vi "mod_control changed.vi"   [LabVIEW 2020, in "niAMT.lvlib"]
uses:
  <vilib>/addons/Modulation/niAMT.lvlib
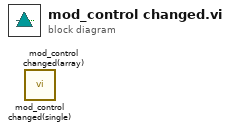
[diagram p0: block diagram]
diagram:
  n1 = call <vilib>:"mod_control changed(single).vi"() -> ()  [unwired: 9 in, 1 out]
  n2 = call <vilib>:"mod_control changed(array).vi"() -> ()  [unwired: 9 in, 1 out]
